vi "Physical Light Emitting Diode Heart Beat PWM.vi"   [LabVIEW 2010]
uses:
  <vilib>/eio/EIONode/EIONode.xnode
  <vilib>/rvi/eio/nirviEIOImplementation/nirviEIOImplementation.xnode
  <vilib>/rvi/eio/common/nirviEmuClasses.ctl
  1.0-Hindbrain Global.vi
  <vilib>/rvi/eio/common/nirviEmuTemplateMethod_noerrors.vi
types:
  T1 = typedef "nirviEmuClasses.ctl" = enum16{"IO Read", "IO Write", "Method", "Property Read", "Property Write"}
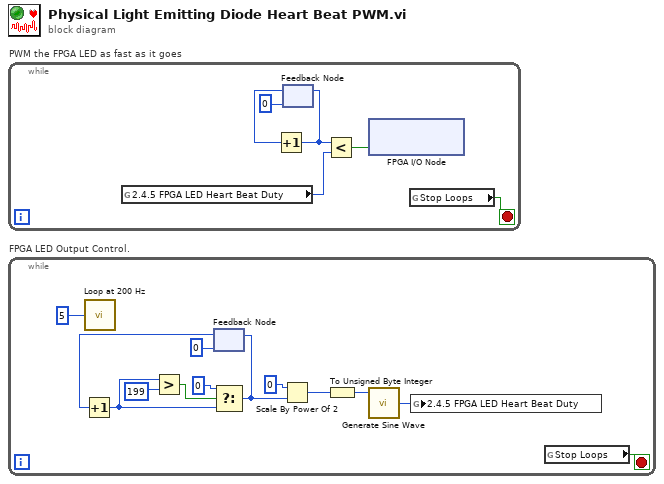
[diagram p0: block diagram]
diagram:
  n1 = while "PWM the FPGA LED as fast as it goes" {
    stop <- w2 stop-if-true
    n2 = global read "1.0-Hindbrain Global.vi" "2.4.5 FPGA LED Heart Beat Duty"() -> (w1:u8)
    n3 = feedback #1(u8 0 ("Heart Beat Duty")) -> (w5:u8)
    n4 = Increment(x=w5) -> (x+1=w4:u8)
    n5 = feedback-in #1(w4) -> ()
    n6 = Less?(x=w4, y=w1) -> (x < y?=w3:bool)
    n7 = xnode "FPGA I/O Node"("FPGA LED"=w3) -> ()  [unwired: 1 in, 1 out]
    n8 = global read "1.0-Hindbrain Global.vi" "Stop Loops"() -> (w2:bool)
  }
  n9 = while "FPGA LED Output Control." {
    stop <- w19 stop-if-true
    n10 = call "Loop at 200 Hz"("Count(mSec)"=u8 5) -> ()  [unwired: 1 out]
    n11 = feedback #2(u16 0 ("Heart Beat Duty")) -> (w29:u16)
    n12 = Increment(x=w29) -> (x+1=w25:u16)
    n13 = Greater?(x=w25, y=u16 199 ("Heart Beat Duty")) -> (0:w26:bool)
    n14 = Select(t=u16 0 ("Heart Beat Duty"), s=w26, f=w25) -> (s? t:f=w23:u16)
    n15 = feedback-in #2(w23) -> ()
    n16 = Scale By Power Of 2(n=0, x=w23) -> (x*2^n=w22:u16)
    n17 = To Unsigned Byte Integer(number=w22) -> (unsigned 8bit integer=w21:u8)
    n18 = call "Generate Sine Wave"("address"=w21) -> ("data out"=w18:u8)  [unwired: 8 in]
    n19 = global write "1.0-Hindbrain Global.vi" "2.4.5 FPGA LED Heart Beat Duty"(w18) -> ()
    n20 = global read "1.0-Hindbrain Global.vi" "Stop Loops"() -> (w19:bool)
  }
